vi "Testing Subpanels.vi"(8 "error in (no error)":errorcluster) -> (0 "error out":errorcluster)   [LabVIEW 2017]
doc: "Use this template to build a VI to use as a subVI."
panel:
  in  "stop":bool
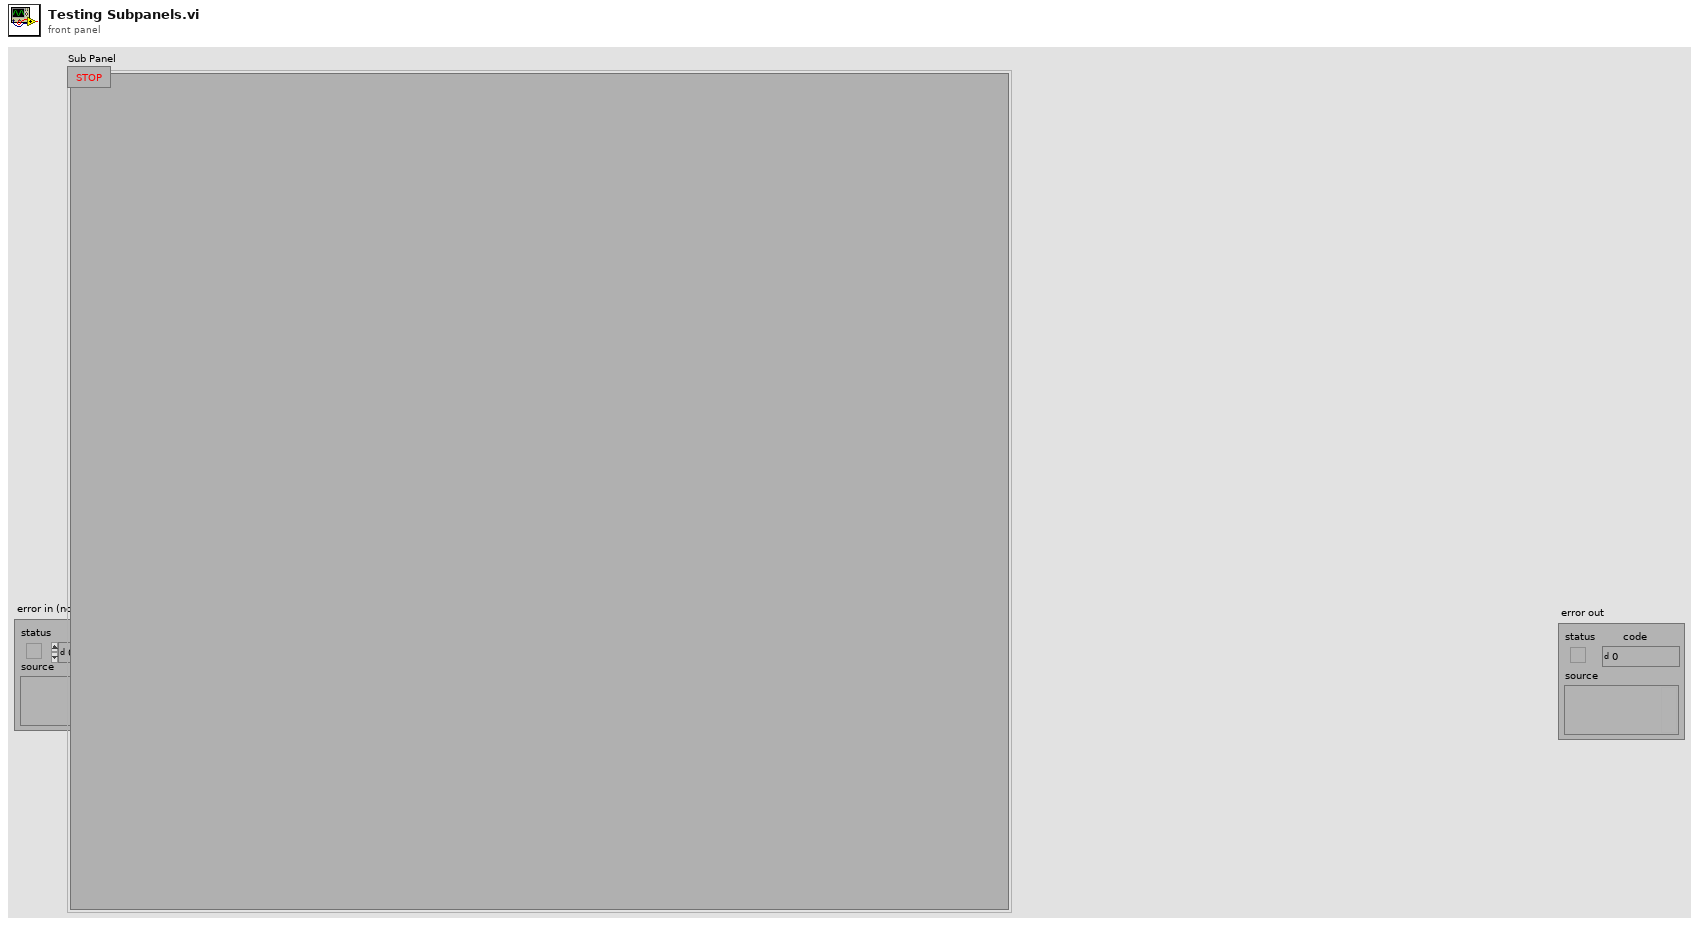
[diagram p1: front panel]
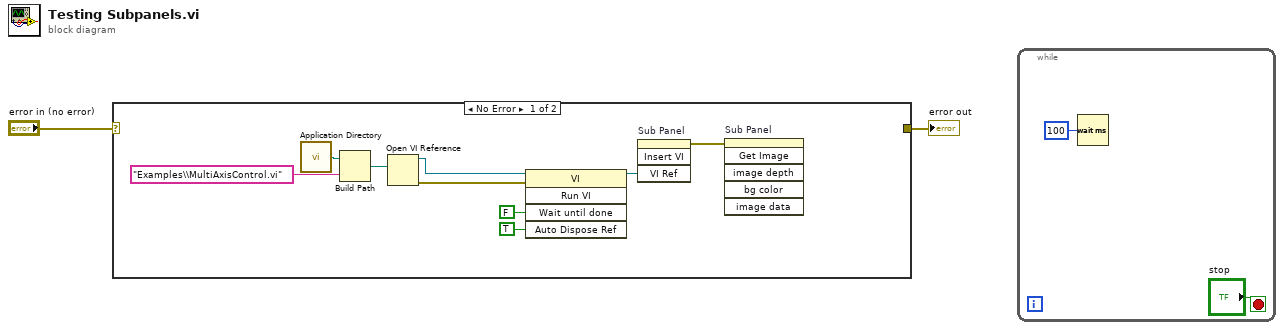
[diagram p0: block diagram]
diagram:
  n1 = case shown="No Error" "error in (no error)" {
    selector: "error in (no error)" -> [_ w12]
    tunnel: [_ w12] -> w1
    frame No Error {
      n2 = call <vilib>:"Application Directory.vi"() -> ("Application Directory"=w9:path)
      n3 = Build Path(base path=w9, name or relative path="Examples\\MultiAxisControl.vi") -> (appended path=w7:path)
      n4 = Open VI Reference(vi path=w7) -> (vi reference=w5:refnum<vi>, error out=w4:errorcluster)  [unwired: 5 in]
      n5 = invoke class="VI" method="Run VI"(reference=w5, error in=w4, "Wait until done"=FALSE ("Wait Until Done"), "Auto Dispose Ref"=TRUE ("Auto Dispose Reference")) -> (reference out=w6:refnum<vi>)  [unwired: 1 in, 4 out]
      n6 = invoke on="Sub Panel" class="SubPanel" method="Insert VI"("VI Ref"=w6) -> (error out=w3:errorcluster)  [unwired: 3 in, 3 out]
      n7 = invoke on="Sub Panel" class="SubPanel" method="Get Image"(error in=w3) -> ()  [unwired: 5 in, 6 out]
    }
    frame Error {
    }
  }
  "error out" <- w1
  n8 = while {
    stop <- "stop" stop-if-true
    n9 = Wait (ms)(milliseconds to wait=u32 100) -> ()  [unwired: 1 out]
  }
